vi "Debug.vi"() -> ()   [LabVIEW 2011, in "Modules.lvlib" / "RSI Module.lvclass"]
uses:
  RSI Module.lvclass
panel:
  in  "Debug?":bool
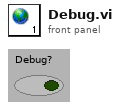
[diagram p1: front panel]
diagram:
